vi "SRV_Execute Multiple W,I Commands.vi"(0 "SRV":refnum<k5>, 7 "Motor Control Commands":T1[](array[typedef]) {"Value" format="%02x"; "Register" format="%02x"; "I2C Address" format="%02x"}, 11 "error in (no error)":errorcluster) -> (4 "SRV Out":refnum<k5>, 10 "Active Array":bool[](array[boolean]), 15 "error out":errorcluster)   [LabVIEW 2014]
doc: "Author: Mike Schultz (LogicPD, Inc)"
uses:
  Motors Config/SRV_Motor Control Command Config.ctl
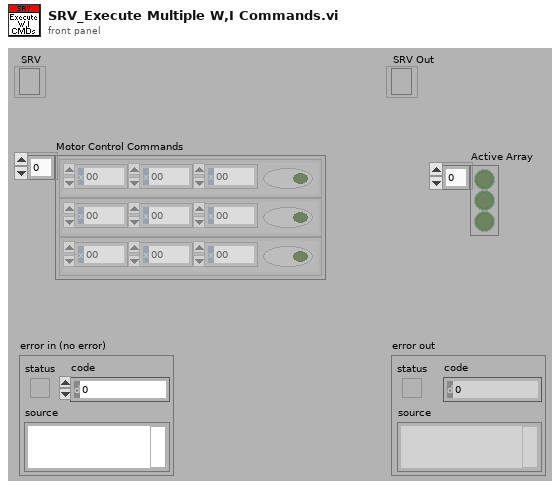
[diagram p1: front panel]
types:
  T1 = typedef "SRV_Motor Control Command Config.ctl" = cluster{"I2C Address":u8, "Register":u8, "Value":u8, "Active":bool}
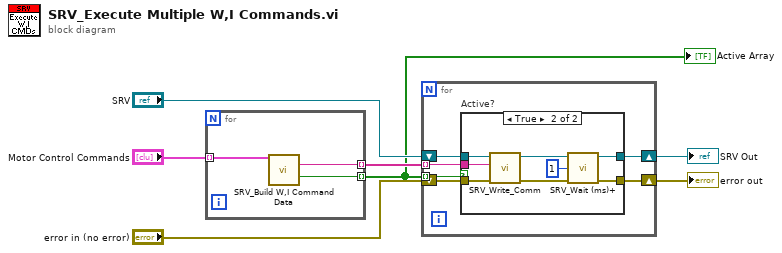
[diagram p0: block diagram]
diagram:
  n1 = for {
    tunnel: "Motor Control Commands" -> [w10] mode=indexing
    tunnel: [w9] -> w2 mode=indexing
    tunnel: [w8] -> w1 mode=indexing
    n2 = call "SRV_Build W,I Command Data.vi"("Motor Control Command"=w10) -> ("Command Data String"=w9:string, "Active"=w8:bool)  [unwired: 12 in, 1 out]
  }
  "Active Array" <- w1
  n3 = for {
    tunnel: w2 -> [w12] mode=indexing
    tunnel: w1 -> [w11] mode=indexing
    shift-right: [w15] -> w6
    shift-left: "SRV" -> [w16]
    shift-right: [w13] -> w4
    shift-left: "error in (no error)" -> [w14]
    n4 = case "Active?" shown="True" w11 {
      tunnel: w16 -> [w17 w25]
      tunnel: [w17 w24] -> w15
      tunnel: w14 -> [w18 w23]
      tunnel: [w18 w20] -> w13
      tunnel: w12 -> [_ w22]
      frame False {
      }
      frame True {
        n5 = call "SRV_Write_Comm.vi"("error in (no error)"=w23, "Command Sent"=w22, "SRV In"=w25) -> ("error out"=w21:errorcluster, "SRV Out"=w24:refnum<k5>)  [unwired: 6 in, 1 out]
        n6 = call "SRV_Wait (ms)+.vi"("milliseconds to wait"=u32 1, "error in (no error)"=w21) -> ("error out"=w20:errorcluster)  [unwired: 12 in, 1 out]
      }
    }
  }
  "SRV Out" <- w6
  "error out" <- w4
